vi "GetValFromFile.vi"(8 "error in (no error)":errorcluster, 9 "regular expression":string, 10 "File path":string, 11 "FW path":path) -> (0 "error out":errorcluster, 3 "extracted value":string)   [LabVIEW 2019, in "LINXx.lvlib"]
uses:
  <vilib>/regexp/Match Regular Expression.xnode
  LINXx.lvlib
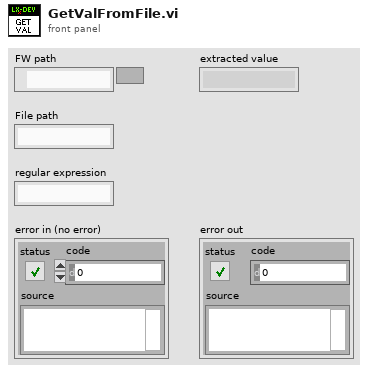
[diagram p1: front panel]
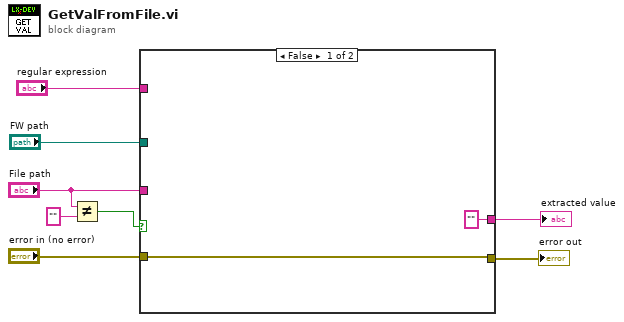
[diagram p0: block diagram]
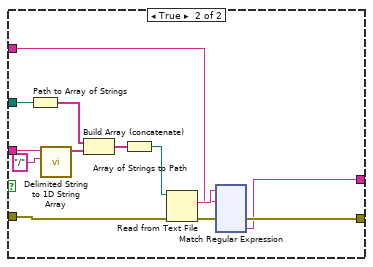
[diagram p2: hidden frame]
diagram:
  n1 = Not Equal?(x="File path", y="") -> (x != y?=w1:bool)
  n2 = case shown="False" w1 {
    tunnel: "File path" -> [_ w22]
    tunnel: "FW path" -> [_ w17]
    tunnel: [w10 w16] -> w7
    tunnel: "error in (no error)" -> [w10 w13]
    tunnel: "regular expression" -> [_ w12]
    tunnel: ["" ("submatch 1") w11] -> w4
    frame False {
    }
    frame True {
      n3 = Path to Array of Strings(0:w17) -> (2:w18:string[])  [unwired: 1 out]
      n4 = call <vilib>:"Delimited String to 1D String Array.vi"("delimiter"="/", "delimited string"=w22) -> ("string array"=w21:string[])  [unwired: 9 in]
      n5 = Build Array (concatenate)(w18, w21) -> (w19:string[])
      n6 = Array of Strings to Path(0:w19) -> (2:w20:path)  [unwired: 1 in]
      n7 = Read from Text File(file (use dialog)=w20, error in=w13) -> (text=w15:string, error out=w14:errorcluster)  [unwired: 2 in, 2 out]
      n8 = xnode "Match Regular Expression"("input string"=w15, "regular expression"=w12, "error in"=w14) -> ("error out"=w16:errorcluster, "submatch 1"=w11:string)  [unwired: 3 in, 4 out]
    }
  }
  "error out" <- w7
  "extracted value" <- w4
